vi "calculate_histogram.vi"(8 "error in (no error)":errorcluster, 9 "# bins (100)":i32=100, 10 "# std deviations for histogram width (1)":dbl=1.0, 11 "2D arr Intensity Graph":dbl[][](array[numeric])=array402x480[192960 elements]) -> (0 "error out":errorcluster, 1 "standard deviation":dbl format="%0.2f", 2 "mean":dbl format="%0.2f", 3 "Histogram Graph":T1(graph))   [LabVIEW 2016]
uses:
  <vilib>/Analysis/NI_AALPro.lvlib
  <vilib>/Analysis/NI_AALBase.lvlib
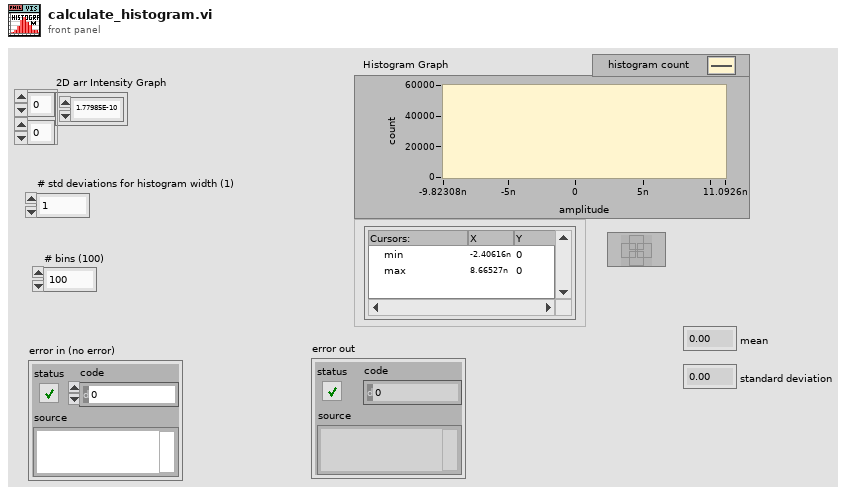
[diagram p1: front panel]
types:
  T1 = cluster{"X Values":dbl[], "Histogram: h(x)":i32[]}
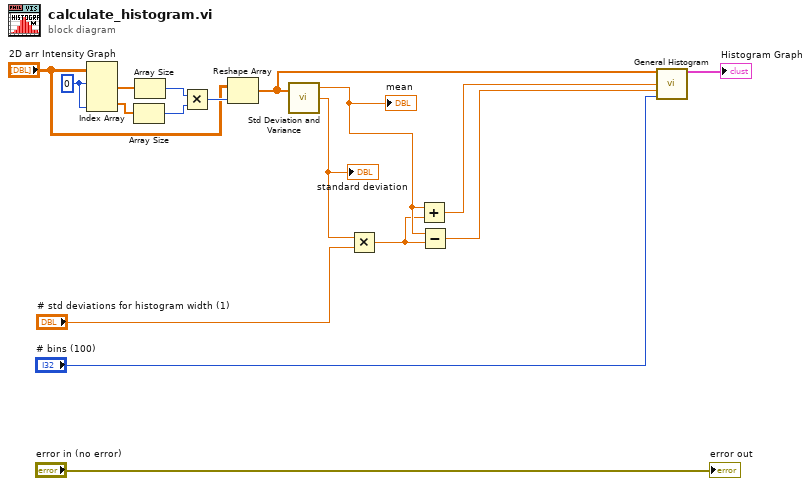
[diagram p0: block diagram]
diagram:
  w10 = 0 ("index (row)")
  n1 = Index Array(array="2D arr Intensity Graph", index (row) #1=w10, index (col) #2=w10) -> (element #1=w11:dbl[], element #2=w9:dbl[])  [unwired: 2 in]
  n2 = Array Size(array=w9) -> (size(s)=w2:i32)
  n3 = Array Size(array=w11) -> (size(s)=w3:i32)
  n4 = Multiply(x=w3, y=w2) -> (x*y=w8:i32)
  n5 = Reshape Array("2D arr Intensity Graph", w8) -> (w4:dbl[])
  n6 = call <vilib>:"Std Deviation and Variance.vi"("X"=w4) -> ("mean"=w17:dbl, "standard deviation"=w14:dbl)  [unwired: 1 in, 1 out]
  "mean" <- w17
  "standard deviation" <- w14
  n7 = Multiply(x=w14, y="# std deviations for histogram width (1)") -> (x*y=w12:dbl)
  n8 = Add(x=w17, y=w12) -> (x+y=w16:dbl)
  n9 = Subtract(x=w17, y=w12) -> (x-y=w15:dbl)
  n10 = call <vilib>:"General Histogram.vi"("X"=w4, "max"=w16, "min"=w15, "# bins"="# bins (100)") -> ("Histogram Graph"=→"Histogram Graph":T1)  [unwired: 7 in, 4 out]
  "error out" <- "error in (no error)"
